vi "GV STAGEZasTrigger.vi"() -> ()   [LabVIEW 2017]
panel:
  out "STAGEZasTrig":bool
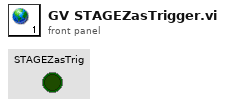
[diagram p1: front panel]
diagram:
